vi "Color pixel (SubVI).vi"(11 "image data":T1) -> (1 "Array":u32[](array[numeric]), 2 "bottom":i16, 3 "right":i16, 4 "image":u8[](array[numeric]))   [LabVIEW 2015]
uses:
  <vilib>/picture/picture.llb/imagedata.ctl
panel:
  in  "Color 3":u32(colorbox)
  in  "Color 2":u32(colorbox)
  in  "Color 1":u32(colorbox)
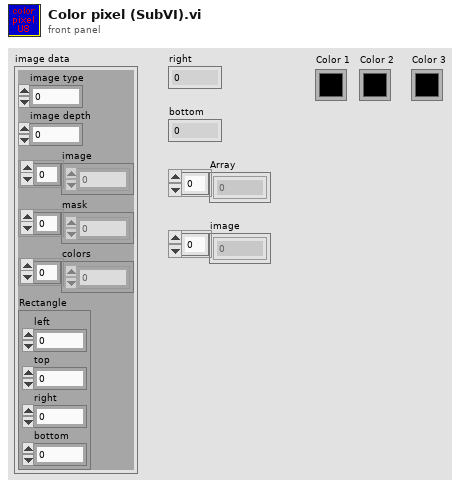
[diagram p1: front panel]
types:
  T1 = typedef "imagedata.ctl" = cluster{"image type":i32, "image depth":i32, "image":u8[], "mask":u8[], "colors":u32[], "Rectangle":cluster{"left":i16, "top":i16, "right":i16, "bottom":i16}}
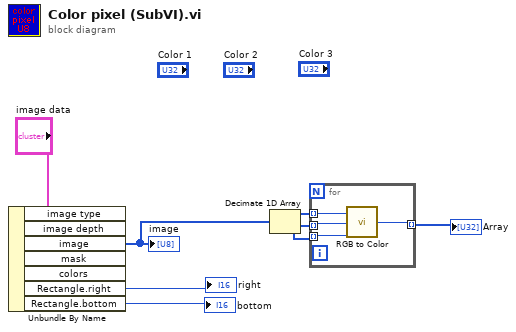
[diagram p0: block diagram]
diagram:
  n1 = Unbundle By Name("image data") -> ("image"=w5:u8[], "Rectangle.right"=→"right":i16, "Rectangle.bottom"=→"bottom":i16)  [unwired: 4 out]
  "image" <- w5
  n2 = Decimate 1D Array(w5) -> (w6:u8[], w7:u8[], w8:u8[])
  n3 = for {
    tunnel: w6 -> [w12] mode=indexing
    tunnel: w7 -> [w11] mode=indexing
    tunnel: w8 -> [w10] mode=indexing
    tunnel: [w9] -> w1 mode=indexing
    n4 = call <vilib>:"RGB to Color.vi"("B"=w10, "G"=w11, "R"=w12) -> ("Color"=w9:u32)
  }
  "Array" <- w1
